vi "get Message By Number.vi"(10 "Message Number":i32, 11 "HMI Messages in":refnum<class "HMI Messages.lvclass">) -> (3 "Message":string)   [LabVIEW 2015, in "HMI Messages.lvclass"]
uses:
  HMI Messages.lvclass
  HMI Messages.lvclass/HMI Messages.ctl
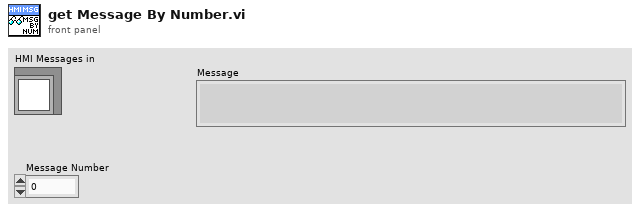
[diagram p1: front panel]
types:
  T1 = typedef "HMI Messages.lvclass/Message Definition.ctl" = cluster{"Number":i32, "Message":string}
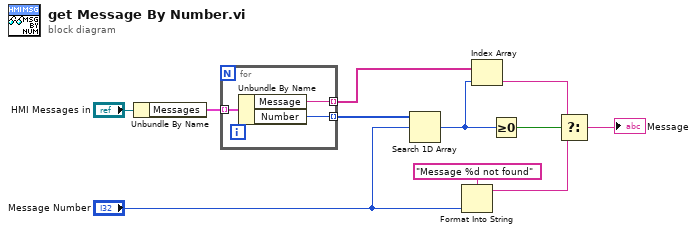
[diagram p0: block diagram]
diagram:
  n1 = Unbundle By Name("HMI Messages in") -> ("Messages"=w10:T1[])
  n2 = for {
    tunnel: w10 -> [w14] mode=indexing
    tunnel: [w13] -> w9 mode=indexing
    tunnel: [w12] -> w5 mode=indexing
    n3 = Unbundle By Name(w14) -> ("Message"=w12:string, "Number"=w13:i32)
  }
  n4 = Search 1D Array(1D array=w9, element="Message Number") -> (index of element=w4:i32)  [unwired: 1 in]
  n5 = Format Into String(format string="Message %d not found", "Message Number") -> (resulting string=w6:string)  [unwired: 2 in, 1 out]
  n6 = Index Array(array=w5, index=w4) -> (element=w3:string)
  n7 = Greater Or Equal To 0?(x=w4) -> (x >= 0?=w8:bool)
  n8 = Select(t=w3, s=w8, f=w6) -> (s? t:f=→"Message":string)
